vi "Left Shift.vi"(8 "Error In":errorcluster, 10 "x":i16, 11 "n":i16) -> (0 "Error Out":errorcluster, 3 "Value":i16)   [LabVIEW 2020, in "LiFingerprint.lvclass"]
uses:
  LiFingerprint.lvclass
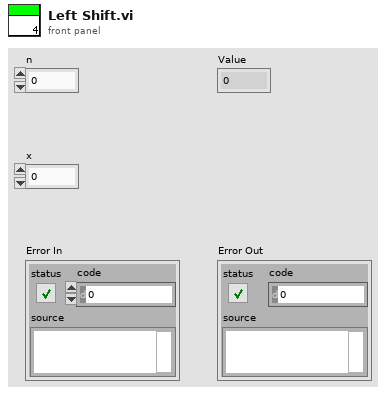
[diagram p1: front panel]
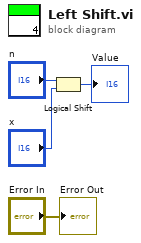
[diagram p0: block diagram]
diagram:
  n1 = Logical Shift(y="n", x="x") -> (x << y=→"Value":i16)
  "Error Out" <- "Error In"
